vi "LVImageDisplay.vi"() -> ()   [LabVIEW 2013]
panel:
  in  "Robot's Address":string="192.168.1.71"
  out "Image Out 3":T1(plugin-control)
  in  "stop":bool
  out "FrameRate":dbl
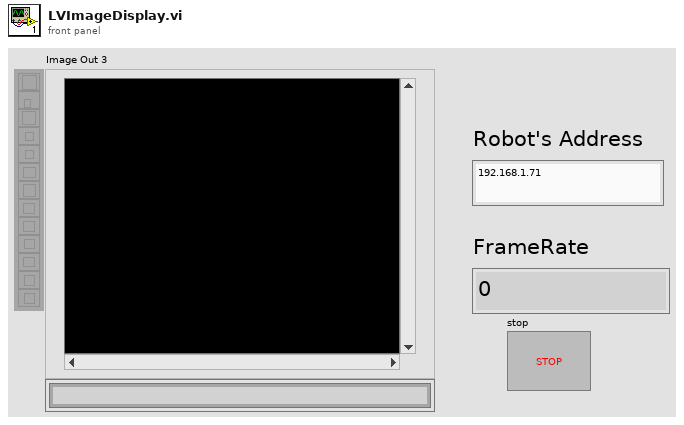
[diagram p1: front panel]
types:
  T1 = typedef "IMAQ Image.ctl" = refnum<image>
  T2 = typedef "Image Type" = u32
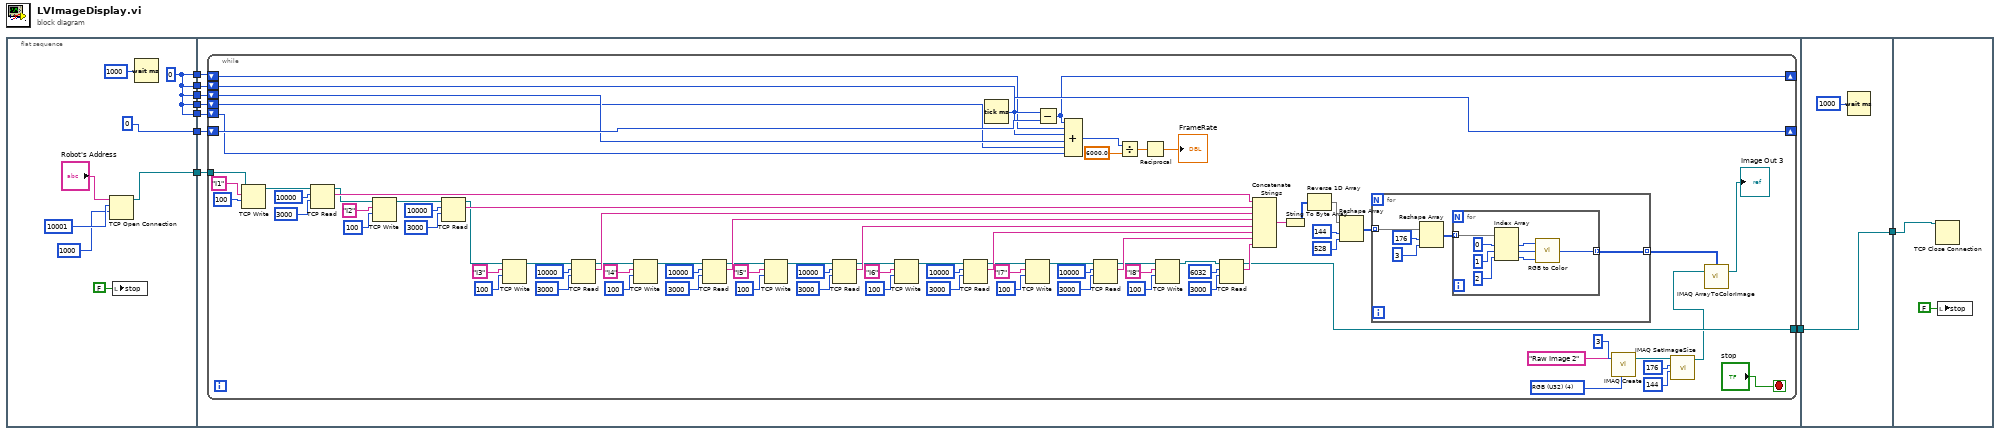
[diagram p0: block diagram]
diagram:
  n1 = flat-sequence {
    tunnel: [w13] -> w9
    tunnel: [0] -> w8
    tunnel: [w10] -> w7
    tunnel: [w10] -> w6
    tunnel: [w10] -> w5
    tunnel: [w10] -> w4
    tunnel: [w10] -> w3
    tunnel: w9 -> [w25]
    tunnel: [w24] -> w2
    tunnel: w8 -> [w23]
    tunnel: w7 -> [w22]
    tunnel: w6 -> [w21]
    tunnel: w5 -> [w20]
    tunnel: w4 -> [w19]
    tunnel: w3 -> [w18]
    tunnel: [w124] -> w1
    tunnel: w2 -> [w124]
    tunnel: w1 -> [w127]
    frame #0 {
      w10 = 0
      n2 = TCP Open Connection(address="Robot's Address", remote port or service name=u16 10001, timeout ms (60000)=1000) -> (connection ID=w13:refnum<k5>)  [unwired: 2 in, 1 out]
      n3 = local write "stop"(FALSE ("stop")) -> ()
      n4 = Wait (ms)(milliseconds to wait=u32 1000) -> ()  [unwired: 1 out]
    }
    frame #1 {
      n5 = while {
        tunnel: w25 -> [w44]
        tunnel: [w43] -> w24
        shift-right: [w40] -> _
        shift-left: w23 -> [w41]
        shift-right: [w35] -> _
        shift-left: w22 -> [w34]
        shift-left: w21 -> [w33]
        shift-left: w20 -> [w32]
        shift-left: w19 -> [w31]
        shift-left: w18 -> [w30]
        stop <- "stop" stop-if-true
        w106 = T2 4 items=["Grayscale (U8)", "Grayscale (I16)", "Grayscale (SGL)", "Complex (CSG)", "RGB (U32)", "HSL (U32)", "RGB (U64)", "Grayscale (U16)"] ("Image Type")
        n6 = TCP Write(connection ID=w44, data in="I1", 9:100 ("timeout ms (25000)")) -> (connection ID out=w47:refnum<k5>)  [unwired: 1 in, 2 out]
        n7 = TCP Read(connection ID=w47, bytes to read=10000, 9:3000 ("timeout ms (25000)")) -> (connection ID out=w49:refnum<k5>, data out=w92:string)  [unwired: 2 in, 1 out]
        n8 = TCP Write(connection ID=w49, data in="I2", 9:100 ("timeout ms (25000)")) -> (connection ID out=w53:refnum<k5>)  [unwired: 1 in, 2 out]
        n9 = TCP Read(connection ID=w53, bytes to read=10000, 9:3000 ("timeout ms (25000)")) -> (connection ID out=w86:refnum<k5>, data out=w93:string)  [unwired: 2 in, 1 out]
        n10 = TCP Write(connection ID=w86, data in="I3", 9:100 ("timeout ms (25000)")) -> (connection ID out=w57:refnum<k5>)  [unwired: 1 in, 2 out]
        n11 = TCP Read(connection ID=w57, bytes to read=10000, 9:3000 ("timeout ms (25000)")) -> (connection ID out=w87:refnum<k5>, data out=w94:string)  [unwired: 2 in, 1 out]
        n12 = TCP Write(connection ID=w87, data in="I4", 9:100 ("timeout ms (25000)")) -> (connection ID out=w64:refnum<k5>)  [unwired: 1 in, 2 out]
        n13 = TCP Read(connection ID=w64, bytes to read=10000, 9:3000 ("timeout ms (25000)")) -> (connection ID out=w88:refnum<k5>, data out=w95:string)  [unwired: 2 in, 1 out]
        n14 = TCP Write(connection ID=w88, data in="I5", 9:100 ("timeout ms (25000)")) -> (connection ID out=w67:refnum<k5>)  [unwired: 1 in, 2 out]
        n15 = TCP Read(connection ID=w67, bytes to read=10000, 9:3000 ("timeout ms (25000)")) -> (connection ID out=w89:refnum<k5>, data out=w96:string)  [unwired: 2 in, 1 out]
        n16 = TCP Write(connection ID=w89, data in="I6", 9:100 ("timeout ms (25000)")) -> (connection ID out=w74:refnum<k5>)  [unwired: 1 in, 2 out]
        n17 = TCP Read(connection ID=w74, bytes to read=10000, 9:3000 ("timeout ms (25000)")) -> (connection ID out=w90:refnum<k5>, data out=w97:string)  [unwired: 2 in, 1 out]
        n18 = Tick Count (ms)() -> (millisecond timer value=w40:u32)
        n19 = TCP Write(connection ID=w90, data in="I7", 9:100 ("timeout ms (25000)")) -> (connection ID out=w77:refnum<k5>)  [unwired: 1 in, 2 out]
        n20 = Subtract(x=w40, y=w41) -> (x-y=w35:u32)
        n21 = Compound Arithmetic op=ADD(w35, w34, w33, w32, w31, w30) -> (w28:u32)
        n22 = TCP Read(connection ID=w77, bytes to read=10000, 9:3000 ("timeout ms (25000)")) -> (connection ID out=w91:refnum<k5>, data out=w98:string)  [unwired: 2 in, 1 out]
        n23 = Divide(x=w28, y=6000.0) -> (x/y=w27:dbl)
        n24 = Reciprocal(x=w27) -> (1/x=→"FrameRate":dbl)
        n25 = TCP Write(connection ID=w91, data in="I8", 9:100 ("timeout ms (25000)")) -> (connection ID out=w84:refnum<k5>)  [unwired: 1 in, 2 out]
        n26 = TCP Read(connection ID=w84, bytes to read=6032, 9:3000 ("timeout ms (25000)")) -> (connection ID out=w43:refnum<k5>, data out=w99:string)  [unwired: 2 in, 1 out]
        n27 = Concatenate Strings(w92, w93, w94, w95, w96, w97, w98, w99) -> (w100:string)
        n28 = String To Byte Array(string=w100) -> (unsigned byte array=w37:u8[])
        n29 = Reverse 1D Array(array=w37) -> (reversed array=w36:u8[])
        n30 = Reshape Array(w36, 144 ("dimension size"), 528 ("dimension size")) -> (w103:u8[][])
        n31 = for {
          tunnel: w103 -> [w113] mode=indexing
          tunnel: [w111] -> w110 mode=indexing
          n32 = Reshape Array(w113, 176 ("dimension size"), 3 ("dimension size")) -> (w112:u8[][])
          n33 = for {
            tunnel: w112 -> [w123] mode=indexing
            tunnel: [w116] -> w111 mode=indexing
            n34 = Index Array(array=w123, index #1=0 ("index"), index #2=1 ("index"), index #3=2 ("index")) -> (element #1=w119:u8, element #2=w118:u8, element #3=w117:u8)
            n35 = call <vilib>:"RGB to Color.vi"("B"=w117, "G"=w118, "R"=w119) -> ("Color"=w116:u32)
          }
        }
        n36 = call "IMAQ Create"("Border Size"=3, "Image Name"="Raw Image 2", "Image Type"=w106) -> ("New Image"=w107:T1)  [unwired: 2 in, 1 out]
        n37 = call "IMAQ SetImageSize"("Y Resolution"=144, "X Resolution"=176, "Image"=w107) -> ("Image Out"=w38:T1)  [unwired: 2 in, 1 out]
        n38 = call "IMAQ ArrayToColorImage"("Image Pixels (U32)"=w110, "Image"=w38) -> ("Image Out"=→"Image Out 3":T1)  [unwired: 3 in, 1 out]
      }
    }
    frame #2 {
      n39 = Wait (ms)(milliseconds to wait=u32 1000) -> ()  [unwired: 1 out]
    }
    frame #3 {
      n40 = TCP Close Connection(connection ID=w127) -> ()  [unwired: 2 in, 2 out]
      n41 = local write "stop"(FALSE ("stop")) -> ()
    }
  }
